vi "Read Endian Match.vi"(8 "error in (no error)":errorcluster, 11 "pcap Parse and Build in":refnum<class "pcap_Parse_Build_CIF.lvclass">) -> (0 "error out":errorcluster, 2 "Endian Match":bool, 3 "pcap Parse and Build out":refnum<class "pcap_Parse_Build_CIF.lvclass">)   [LabVIEW 2021, in "pcap_Parse_Build_CIF.lvclass"]
uses:
  pcap_Parse_Build_CIF.lvclass
  pcap_Parse_Build_CIF.lvclass/pcap_Parse_Build_CIF.ctl
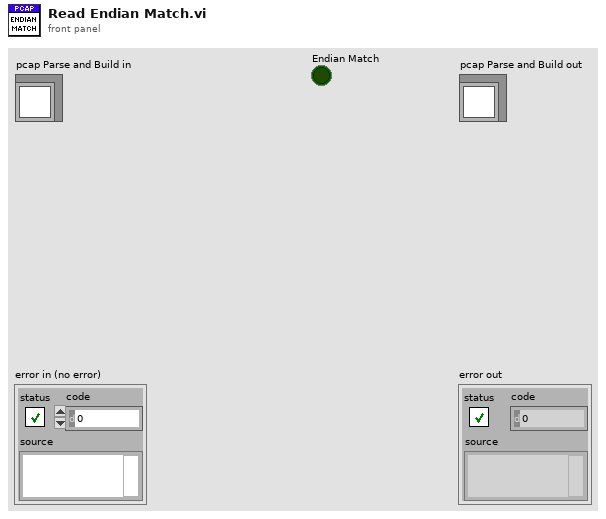
[diagram p1: front panel]
types:
  T1 = typedef "DataTypes_CIF_U.lvlib/Endian.ctl" = enum16{"Little Endian", "Big Endian"}
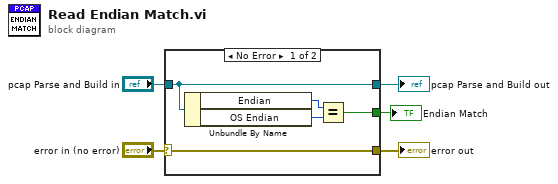
[diagram p0: block diagram]
diagram:
  n1 = case shown="No Error" "error in (no error)" {
    selector: "error in (no error)" -> [w10 w11]
    tunnel: [w10 w11] -> w4
    tunnel: [w9 w12] -> w2
    tunnel: "pcap Parse and Build in" -> [w9 w12]
    tunnel: [w6 _] -> w1
    frame No Error {
      n2 = Unbundle By Name(w9) -> ("Endian"=w8:T1, "OS Endian"=w7:T1)
      n3 = Equal?(x=w8, y=w7) -> (x = y?=w6:bool)
    }
    frame Error {
    }
  }
  "error out" <- w4
  "pcap Parse and Build out" <- w2
  "Endian Match" <- w1
